vi "Icon_Find PixelValue at Point.vi"(9 "Point":T1, 11 "Picture":picture) -> (3 "Color Box Out":u32(colorbox))   [LabVIEW 2021]
uses:
  <vilib>/Utility/miscctls.llb/LVPositionTypeDef.ctl
  vi.lib/LabVIEW Icon API/lv_icon/lv_icon.lvlib
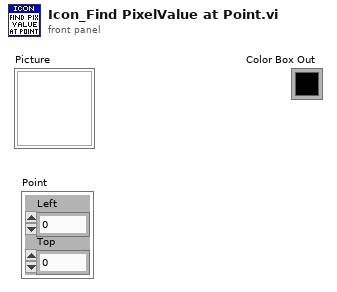
[diagram p1: front panel]
types:
  T1 = typedef "LVPositionTypeDef.ctl" = cluster{"Left":i32, "Top":i32}
  T2 = cluster{"left":i16, "top":i16, "right":i16, "bottom":i16}
  T3 = typedef "imagedata.ctl" = cluster{"image type":i32, "image depth":i32, "image":u8[], "mask":u8[], "colors":u32[], "Rectangle":cluster{"left":i16, "top":i16, "right":i16, "bottom":i16}}
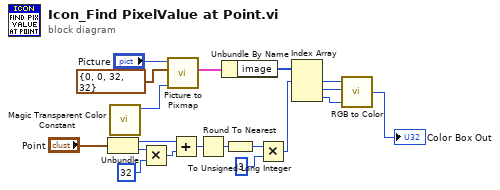
[diagram p0: block diagram]
diagram:
  n1 = Unbundle("Point") -> ("Left"=w12:i32, "Top"=w5:i32)
  n2 = call "Magic Transparent Color Constant.vi"() -> ("Magic transparent color constant"=w3:u32)  [unwired: 11 out]
  n3 = Multiply(x=w5, y=32) -> (x*y=w4:i32)
  n4 = call <vilib>:"Picture to Pixmap.vi"("Background Color"=w3, "rect"=T2 {"left"=0, "top"=0, "right"=32, "bottom"=32}, "picture"="Picture") -> ("image data"=w13:T3)  [unwired: 1 in, 7 out]
  n5 = Add(x=w12, y=w4) -> (x+y=w9:i32)
  n6 = Round To Nearest(number=w9) -> (nearest integer value=w8:i32)
  n7 = Unbundle By Name(w13) -> ("image"=w14:u8[])
  n8 = To Unsigned Long Integer(number=w8) -> (unsigned 32bit integer=w11:u32)
  n9 = Multiply(x=w11, y=u32 3) -> (x*y=w15:u32)
  n10 = Index Array(array=w14, index #1=w15) -> (element #1=w16:u8, element #2=w17:u8, element #3=w18:u8)  [unwired: 2 in]
  n11 = call <vilib>:"RGB to Color.vi"("B"=w18, "G"=w17, "R"=w16) -> ("Color"=→"Color Box Out":u32)
